vi "Tester_Laser80Calc160.vi"() -> ()   [LabVIEW 2012]
uses:
  <vilib>/Platform/TimedLoop/XDataNode/timing_clust.ctl
  <vilib>/Platform/TimedLoop/XDataNode/nitl_modes.ctl
  <vilib>/Platform/TimedLoop/XDataNode/wakeup.ctl
  <vilib>/rvi/Emulation/niFpgaSctlEmulationRegisterWithScheduler.vi
  <vilib>/rvi/eio/common/nirviEmuTemplateMethod_errors.vi
  <vilib>/rvi/Emulation/niFpgaSctlEmulationScheduler.vi
  <vilib>/rvi/FIFO/Fifo_Resource/nirvififoEmulationSetSize.vi
  <vilib>/rvi/DataTransferAndStorage/Container/Common/niFpgaContainerGetUniqueNameForEmu.vi
  <vilib>/rvi/errors/niFpgaSetErrorForExecOnDevCompSimple.vi
  <vilib>/rvi/eio/common/nirviEmuReportErrorAndStop.vi
  <vilib>/rvi/Emulation/niFpgaSctlEmulationFifoFullMgr.vi
  <vilib>/rvi/Emulation/niFpgaSctlEmulationResourceMgr.vi
  <vilib>/rvi/interface/RandomDataEmulation/nirviRandomDataFPGAFIFO.vi
  <vilib>/rvi/interface/RandomDataEmulation/niFpgaRandomDataHandleErrors.vi
  <vilib>/rvi/Emulation/niFpgaSctlEmulationGlobalWrite.vi
  <vilib>/Platform/TimedLoop/XDataNode/XDataNode.xnode
  <vilib>/eio/EIONode/EIONode.xnode
  <vilib>/rvi/DataTransferAndStorage/Container/XNode/niFpgaContainer.xnode
  <vilib>/rvi/FIFO/Fifo_Resource/nirvififoEmulationClear.vi
  <vilib>/rvi/FIFO/Fifo_Resource/nirvififoEmulationWrite.vi
  <vilib>/rvi/FIFO/Fifo_Resource/nirvififoEmulationRead.vi
  <vilib>/rvi/interface/RandomDataEmulation/nirviRandomDataFpgaReadWriteTemplate.vi
  <vilib>/Platform/TimedLoop/XDataNode/XDNodeRunTimeDep.lvlib
panel:
  out "ToHostAreas FIFO Overflow":bool
  out "ToHostArea1LaserRaw FIFO Overflow":bool
  out "ToHostCh1Raw FIFO Overflow":bool
  out "ToHost FIFO Overflow A1Ch2":bool
  in  "Switch for":i32=6 caption="Requested pixels"
  in  "Laser bitslip":bool
  in  "Laser delay inc":bool
  in  "Samples per pixel Acq A2":u16=10000 caption="Samples per pixel Acq"
  in  "Samples per pixel Acq A1":u16=10000 caption="Samples per pixel Acq"
  in  "Requested pixels A2":u32=100000 caption="Requested pixels"
  in  "Samples per pixel A2":u16=10000 caption="Samples per pixel"
  out "Acquiring":bool
  in  "Wait for trigger":bool
  in  "Acquire continuously":bool=TRUE
  in  "Requested pixels A1":u32=100000 caption="Requested pixels"
  in  "Clear Interloop FIFO":bool
  out "Interloop FIFO overflow":bool
  in  "Samples per pixel A1":u16=10000 caption="Samples per pixel"
  in  "Acquire":bool
  out "Interloop FIFO timeout":bool
  in  "Commit":bool
  out "Xpoint_Switch_Ready":bool
  in  "Xpoint_Switch_Write":bool
  in  "Clock Source":u8(ring)=3 items=["Tristate"=0, "Sync Clock (PXIe only)"=2, "Adapter Module Onboard Clock"=3, "Strobe from Crosspoint Switch"=4, "Strobe Bypass"=5]
  in  "Onboard_Clock_Write":bool
  in  "Onboard_Clock_Write_Data":u16
  out "Onboard_Clock_Ready":bool
  in  "Acq_Reset":bool
  # "6587 IO module configuration"
  # "Tester - Laser80MHz/Calculate 160MHz"
  # "Acquisition control"
  # "Area 1"
  # "Area 2"
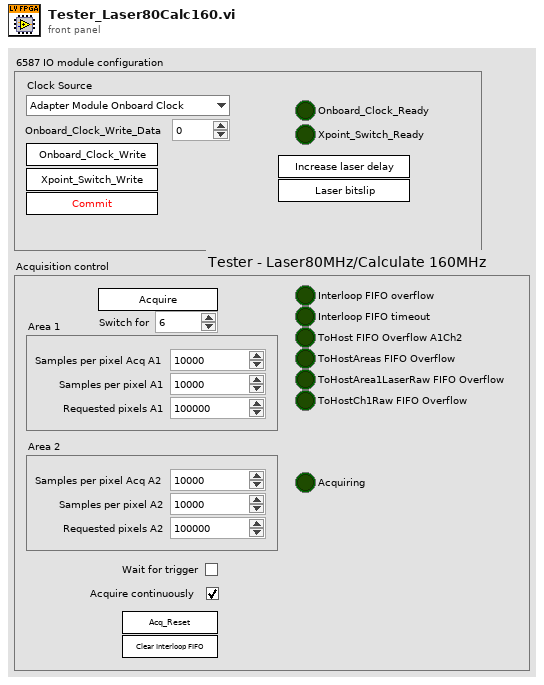
[diagram p1: front panel]
types:
  T1 = typedef "XDNodeRunTimeDep.lvlib/timing_clust.ctl" = cluster{"Expected End [f-1]":u64, "Actual End [f-1]":u64, "Finished Late? [f-1]":bool, "Expected End [i-1]":u64, "Actual End [i-1]":u64, "Finished Late? [i-1]":bool, "Expected Start [i]":u64, "Actual Start [i]":u64, "Expected Start [f]":u64, "Actual Start [f]":u64, "Source Name":string, "Structure Name":string, "Period":i64, "Deadline":i64, "Offset":i64, "Start":i64, "Priority":i32, "Timeout":i32, "Mode":T2, "Wakeup Reason":T3, "Error":errorcluster, "Source Type":string, "Secondary Source Type":string, "Global End Time":u64, "Global Start Time":u64, "Frame Duration":u64, "Iteration Duration":u64, "Assigned CPU":i32, "I/O Scan Engine Mode":u32}
  T2 = typedef "XDNodeRunTimeDep.lvlib/nitl_modes.ctl" = enum32{"No Change", "Process missed periods, maintain original phase", "Discard missed periods, maintain original phase", "Process missed periods, ignore original phase", "Discard missed periods, ignore original phase"}
  T3 = typedef "XDNodeRunTimeDep.lvlib/wakeup.ctl" = enum32{"Normal", "Aborted", "Asynchronous wakeup", "Timing source error", "Timed loop error", "Timeout"}
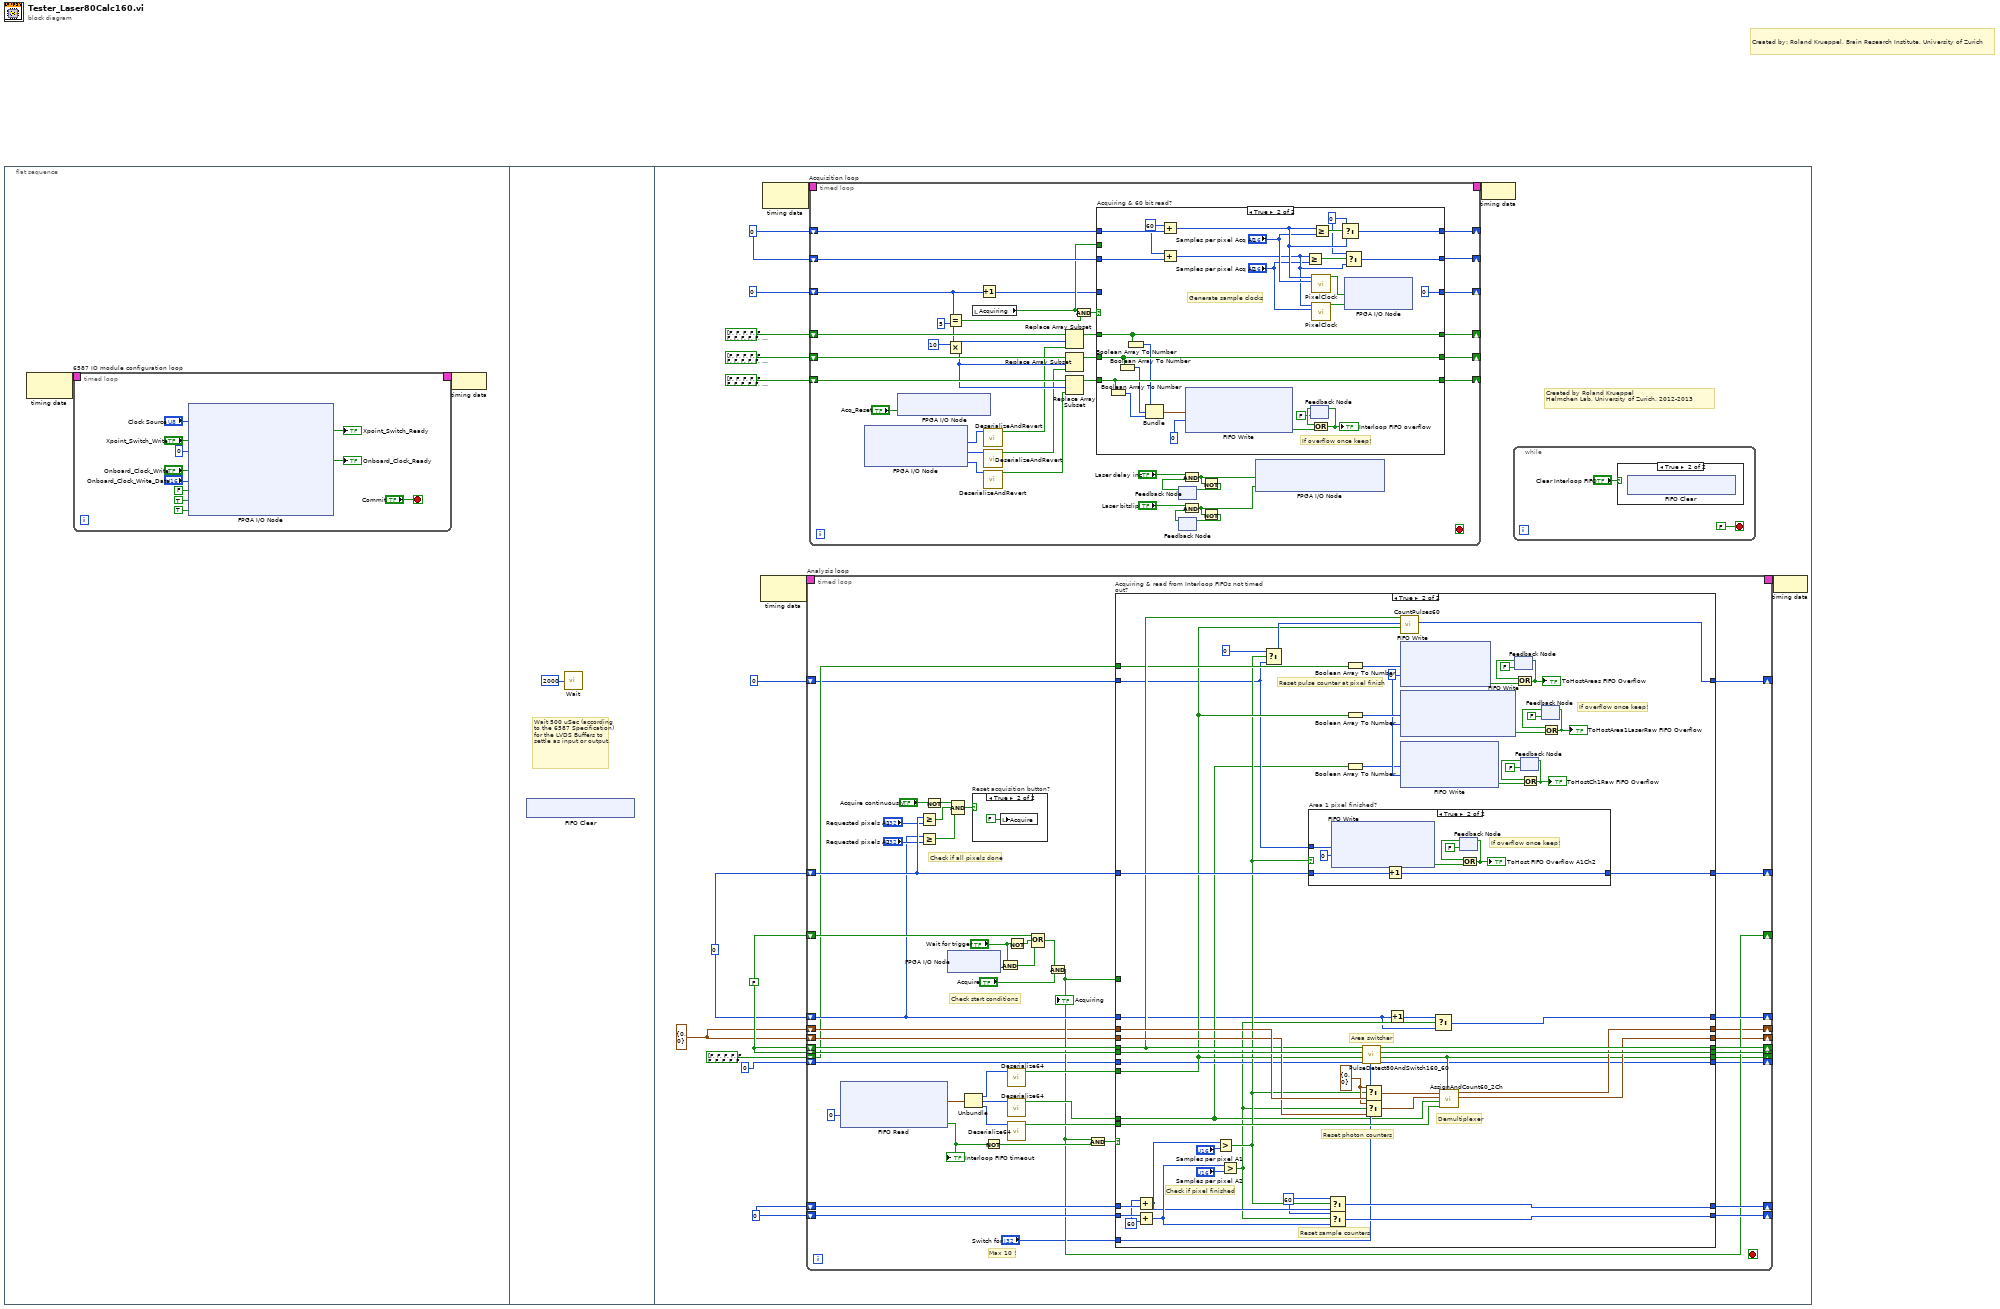
[diagram p0: block diagram]
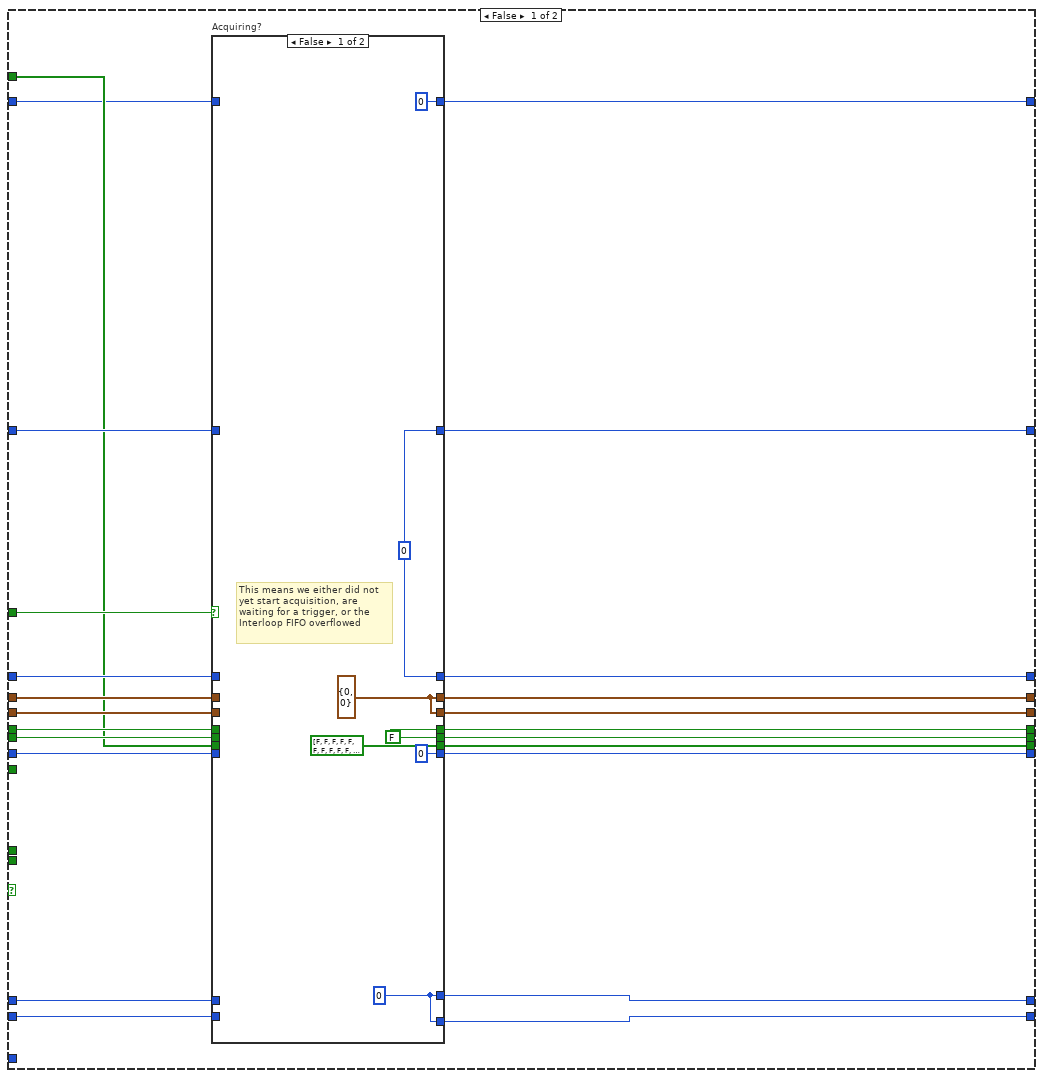
[diagram p4: hidden frame]
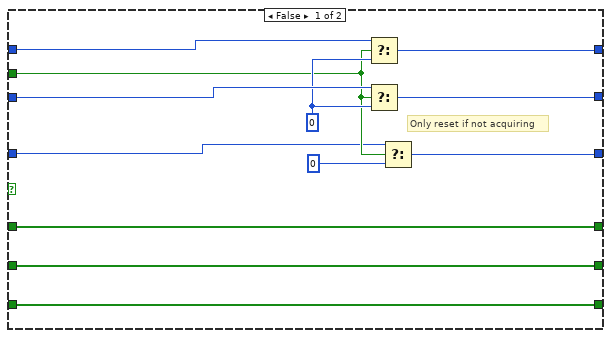
[diagram p7: hidden frame]
diagram:
  # "Created by: Roland Krueppel, Brain Research Institute, University of Zurich"
  n1 = flat-sequence {
    frame #0 {
      n2 = node-c288() -> (w2:T1)  [unwired: 1 in]
      n3 = timed-loop "6587 IO module configuration loop" {
        timing: w2 -> [_]
        timing-out: [_] -> w1
        stop <- "Commit" stop-if-true
        n4 = xnode "FPGA I/O Node"("IO Module\\Acq_IO_Clock_Source"="Clock Source", "IO Module\\Xpoint_Switch_Write"="Xpoint_Switch_Write", "IO Module\\LVDS_Data_Dir"=u16 0 ("IO Module\\LVDS_Data_Dir"), "IO Module\\Onboard_Clock_Write"="Onboard_Clock_Write", "IO Module\\Onboard_Clock_Write_Data"="Onboard_Clock_Write_Data", "IO Module\\SE_PFI0_WE"=FALSE ("IO Module\\SE_PFI0_WE"), "IO Module\\SE_PFI1_WE"=TRUE ("IO Module\\SE_PFI1_WE"), "IO Module\\SE_PFI2_WE"=TRUE ("IO Module\\SE_PFI2_WE")) -> ("IO Module\\Xpoint_Switch_Ready"=→"Xpoint_Switch_Ready":bool, "IO Module\\Onboard_Clock_Ready"=→"Onboard_Clock_Ready":bool)  [unwired: 10 in, 10 out]
      }
      n5 = node-c288(w1) -> ()
    }
    frame #1 {
      # "Wait 500 uSec (according to the 6587 Specification) for the LVDS Buffers to settle as input or output."
      n6 = xnode "FIFO Clear"() -> ()  [unwired: 1 in, 1 out]
      n7 = call "Wait"("Count(uSec)"=u32 2000) -> ()  [unwired: 1 out]
    }
    frame #2 {
      w19 = u16 0 ("t")
      w23 = cluster{u16, u16} {0, 0} ("output cluster")
      w24 = u16 0
      w25 = u32 0 ("Cycle counter out")
      w26 = FALSE ("Last laser bit out")
      # "Created by Roland Krueppel\nHelmchen Lab, University of Zurich, 2012-2013"
      n8 = node-c288() -> (w32:T1)  [unwired: 1 in]
      n9 = node-c288() -> (w34:T1)  [unwired: 1 in]
      n10 = timed-loop "Analysis loop" {
        timing: w32 -> [_]
        timing-out: [_] -> w31
        shift-right: [w82] -> _
        shift-left: w26 -> [w85]
        shift-right: [w84] -> _
        shift-left: w26 -> [w83]
        shift-right: [w58] -> _
        shift-left: w19 -> [w81]
        shift-right: [w56] -> _
        shift-left: w25 -> [w80]
        shift-right: [w54] -> _
        shift-left: w26 -> [w69]
        shift-right: [w57] -> _
        shift-left: w19 -> [w64]
        shift-right: [w55] -> _
        shift-left: w25 -> [w62]
        shift-right: [w45] -> _
        shift-left: w23 -> [w47]
        shift-right: [w44] -> _
        shift-left: w23 -> [w46]
        shift-right: [w43] -> _
        shift-left: bool[] [FALSE, FALSE, FALSE, FALSE, FALSE, FALSE, FALSE, FALSE, FALSE, FALSE, FALSE, FALSE, FALSE, FALSE, FALSE, FALSE, FALSE, FALSE, FALSE, FALSE, FALSE, FALSE, FALSE, FALSE, FALSE, FALSE, FALSE, FALSE, FALSE, FALSE, FALSE, FALSE, FALSE, FALSE, FALSE, FALSE, FALSE, FALSE, FALSE, FALSE, FALSE, FALSE, FALSE, FALSE, FALSE, FALSE, FALSE, FALSE, FALSE, FALSE, FALSE, FALSE, FALSE, FALSE, FALSE, FALSE, FALSE, FALSE, FALSE, FALSE] ("Area bits out") -> [w42]
        shift-right: [w41] -> _
        shift-left: u16 0 ("New pulse count") -> [w40]
        shift-right: [w39] -> _
        shift-left: 0 ("Fill after last") -> [w38]
        stop <- _ stop-if-true
        # "Max 10 !"
        # "Check start conditions"
        # "Check if all pixels done"
        n11 = xnode ("FIFO Read")("Timeout"=0) -> ("Element"=w51:cluster{"Laser":u64, "Ch0":u64, "Ch1":u64}, "Timed Out?"=w52:bool)  [unwired: 1 in, 1 out]
        "Interloop FIFO timeout" <- w52
        n12 = Greater Or Equal?(x=w80, y="Requested pixels A1") -> (x >= y?=w60:bool)
        n13 = Greater Or Equal?(x=w62, y="Requested pixels A2") -> (x >= y?=w59:bool)
        n14 = Not(x="Acquire continuously") -> (.not. x?=w61:bool)
        n15 = xnode "FPGA I/O Node"() -> ("TriggerIn"=w75:bool)  [unwired: 1 in, 1 out]
        n16 = Compound Arithmetic op=AND(w61, w60, w59) -> (w77:bool)
        n17 = Unbundle(w51) -> ("Laser"=w50:u64, "Ch0"=w49:u64, "Ch1"=w48:u64)
        n18 = case "Reset acquisition button?" shown="True" w77 {
          frame False {
          }
          frame True {
            n19 = local write "Acquire"(FALSE ("Acquire")) -> ()
          }
        }
        n20 = Not(x=w52) -> (.not. x?=w70:bool)
        n21 = And(x="Wait for trigger", y=w75) -> (x .and. y?=w72:bool)
        n22 = call "Deserialize64.vi"("U64 input"=w50) -> ("60bit output"=w67:bool[])  [unwired: 10 in]
        n23 = call "Deserialize64.vi"("U64 input"=w49) -> ("60bit output"=w66:bool[])  [unwired: 10 in]
        n24 = call "Deserialize64.vi"("U64 input"=w48) -> ("60bit output"=w65:bool[])  [unwired: 10 in]
        n25 = Not(x="Wait for trigger") -> (.not. x?=w73:bool)
        n26 = Compound Arithmetic op=OR(w69, w73, w72) -> (w71:bool)
        n27 = And(x=w71, y="Acquire") -> (x .and. y?=w54:bool)
        "Acquiring" <- w54
        n28 = And(x=w54, y=w70) -> (x .and. y?=w68:bool)
        n29 = case "Acquiring & read from Interloop FIFOs not timed out?" shown="True" w68 {
          tunnel: w85 -> [w104 w171]
          tunnel: w47 -> [w108 w168]
          tunnel: [w103 w170] -> w84
          tunnel: w83 -> [w105 w159]
          tunnel: [w102 w169] -> w82
          tunnel: w81 -> [w107 w183]
          tunnel: w80 -> [w106 w179]
          tunnel: w67 -> [_ w152]
          tunnel: w66 -> [_ w145]
          tunnel: w54 -> [w109 _]
          tunnel: w65 -> [_ w164]
          tunnel: w64 -> [w96 w181]
          tunnel: w62 -> [w99 w140]
          tunnel: [w97 w173] -> w58
          tunnel: [w95 w175] -> w57
          tunnel: [w101 w162] -> w45
          tunnel: [w100 w178] -> w56
          tunnel: [w98 w141] -> w55
          tunnel: w46 -> [w94 w166]
          tunnel: [w93 w161] -> w44
          tunnel: [w91 w160] -> w43
          tunnel: w42 -> [w92 w154]
          tunnel: [w89 w158] -> w41
          tunnel: w40 -> [w90 w150]
          tunnel: [w87 w149] -> w39
          tunnel: w38 -> [w88 w148]
          tunnel: "Switch for" -> [_ w147]
          frame False {
            n30 = case "Acquiring?" shown="False" w109 {
              tunnel: w108 -> [_ w125]
              tunnel: w107 -> [_ w122]
              tunnel: w106 -> [_ w124]
              tunnel: w105 -> [_ w127]
              tunnel: w104 -> [_ w126]
              tunnel: [w116 w127] -> w103
              tunnel: [w116 w126] -> w102
              tunnel: [w114 w125] -> w101
              tunnel: [w115 w124] -> w100
              tunnel: w99 -> [_ w123]
              tunnel: [w115 w123] -> w98
              tunnel: [w113 w122] -> w97
              tunnel: [w113 w121] -> w95
              tunnel: w96 -> [_ w121]
              tunnel: w94 -> [_ w120]
              tunnel: [w114 w120] -> w93
              tunnel: w92 -> [_ w119]
              tunnel: [bool[] [FALSE, FALSE, FALSE, FALSE, FALSE, FALSE, FALSE, FALSE, FALSE, FALSE, FALSE, FALSE, FALSE, FALSE, FALSE, FALSE, FALSE, FALSE, FALSE, FALSE, FALSE, FALSE, FALSE, FALSE, FALSE, FALSE, FALSE, FALSE, FALSE, FALSE, FALSE, FALSE, FALSE, FALSE, FALSE, FALSE, FALSE, FALSE, FALSE, FALSE, FALSE, FALSE, FALSE, FALSE, FALSE, FALSE, FALSE, FALSE, FALSE, FALSE, FALSE, FALSE, FALSE, FALSE, FALSE, FALSE, FALSE, FALSE, FALSE, FALSE] ("Area bits out") w119] -> w91
              tunnel: w90 -> [_ w118]
              tunnel: [u16 0 ("New pulse count") w118] -> w89
              tunnel: w88 -> [_ w117]
              tunnel: [0 ("Fill after last") w117] -> w87
              frame False {
                w114 = cluster{u16, u16} {0, 0} ("output cluster")
                w115 = u32 0 ("Cycle counter out")
                w113 = u16 0
                w116 = FALSE ("Last laser bit out")
                # "This means we either did not\nyet start acquisition, are\nwaiting for a trigger, or the\nInterloop FIFO overflowed"
              }
              frame True {
                # "This means we are\nreading faster here\nthan acquiring in\nAcquisition loop\n-> keep all values"
              }
            }
          }
          frame True {
            w146 = 0 ("Timeout")
            w163 = cluster{u16, u16} {0, 0} ("t")
            w172 = u16 60 ("t")
            w180 = u16 60
            # "If overflow once keep!"
            # "Reset pulse counter at pixel finish"
            # "Demultiplexer"
            # "Reset photon counters"
            # "Area switcher"
            # "Check if pixel finished"
            # "Reset sample counters"
            n31 = Add(x=w180, y=w183) -> (x+y=w174:u16)
            n32 = Add(x=w181, y=w180) -> (x+y=w176:u16)
            n33 = Greater?(x=w174, y="Samples per pixel A1") -> (0:w151:bool)
            n34 = Greater?(x=w176, y="Samples per pixel A2") -> (0:w143:bool)
            n35 = Select(t=u16 0, s=w151, f=w150) -> (s? t:f=w157:u16)
            n36 = case "Area 1 pixel finished?" shown="True" w151 {
              tunnel: w179 -> [w184 w192]
              tunnel: [w184 w191] -> w178
              tunnel: w150 -> [_ w190]
              frame False {
              }
              frame True {
                # "If overflow once keep!"
                n37 = xnode ("FIFO Write")("Element"=w190, "Timeout"=0) -> ("Timed Out?"=w186:bool)  [unwired: 1 in, 1 out]
                n38 = Increment(x=w192) -> (x+1=w191:u32)
                n39 = feedback #1(FALSE) -> (w188:bool)
                n40 = Or(x=w188, y=w186) -> (x .or. y?=w185:bool)
                "ToHost FIFO Overflow A1Ch2" <- w185
                n41 = feedback-in #1(w185) -> ()
              }
            }
            n42 = Select(t=w172, s=w151, f=w174) -> (s? t:f=w173:u16)
            n43 = Select(t=w172, s=w143, f=w176) -> (s? t:f=w175:u16)
            n44 = Boolean Array To Number(Boolean array=w154) -> (number=w155:u64)
            n45 = Boolean Array To Number(Boolean array=w152) -> (number=w153:u64)
            n46 = Boolean Array To Number(Boolean array=w145) -> (number=w144:u64)
            n47 = call "PulseDetect80AndSwitch160_60.vi"("Switch for"=w147, "Fill from last"=w148, "Laser bits in"=w152, "Last area in"=w171, "Last laser bit in"=w159) -> ("Fill after last"=w149:i32, "Area bits out"=w160:bool[], "New last area out"=w169:bool, "New last laser bit out"=w170:bool)  [unwired: 3 in]
            n48 = Select(t=w163, s=w151, f=w168) -> (s? t:f=w167:cluster{u16, u16})
            n49 = Select(t=w163, s=w143, f=w166) -> (s? t:f=w165:cluster{u16, u16})
            n50 = Increment(x=w140) -> (x+1=w142:u32)
            n51 = call "CountPulses60.vi"("60bit input"=w152, "Previous pulse count"=w157, "Last sample"=w159) -> ("New pulse count"=w158:u16)  [unwired: 7 in, 1 out]
            n52 = xnode ("FIFO Write")("Element"=w155, "Timeout"=w146) -> ("Timed Out?"=w129:bool)  [unwired: 1 in, 1 out]
            n53 = xnode ("FIFO Write")("Element"=w153, "Timeout"=w146) -> ("Timed Out?"=w133:bool)  [unwired: 1 in, 1 out]
            n54 = xnode ("FIFO Write")("Element"=w144, "Timeout"=w146) -> ("Timed Out?"=w136:bool)  [unwired: 1 in, 1 out]
            n55 = Select(t=w142, s=w143, f=w140) -> (s? t:f=w141:u32)
            n56 = call "AssignAndCount60_2Ch.vi"("Area bits in"=w160, "PMT bits Ch2 in"=w164, "PMT bits Ch1 in"=w145, "Photon counters area 2 in"=w165, "Photon counters area 1 in"=w167) -> ("Photon counters area 2 out"=w161:cluster{u16, u16}, "Photon counters area 1 out"=w162:cluster{u16, u16})  [unwired: 5 in]
            n57 = feedback #2(FALSE) -> (w128:bool)
            n58 = Or(x=w128, y=w129) -> (x .or. y?=w130:bool)
            "ToHostAreas FIFO Overflow" <- w130
            n59 = feedback-in #2(w130) -> ()
            n60 = feedback #3(FALSE) -> (w139:bool)
            n61 = Or(x=w139, y=w136) -> (x .or. y?=w137:bool)
            "ToHostCh1Raw FIFO Overflow" <- w137
            n62 = feedback-in #3(w137) -> ()
            n63 = feedback #4(FALSE) -> (w132:bool)
            n64 = Or(x=w132, y=w133) -> (x .or. y?=w134:bool)
            "ToHostArea1LaserRaw FIFO Overflow" <- w134
            n65 = feedback-in #4(w134) -> ()
          }
        }
      }
      n66 = timed-loop "Acquisition loop" {
        timing: w34 -> [_]
        timing-out: [_] -> w33
        shift-right: [w224] -> _
        shift-left: bool[] [FALSE, FALSE, FALSE, FALSE, FALSE, FALSE, FALSE, FALSE, FALSE, FALSE, FALSE, FALSE, FALSE, FALSE, FALSE, FALSE, FALSE, FALSE, FALSE, FALSE, FALSE, FALSE, FALSE, FALSE, FALSE, FALSE, FALSE, FALSE, FALSE, FALSE, FALSE, FALSE, FALSE, FALSE, FALSE, FALSE, FALSE, FALSE, FALSE, FALSE, FALSE, FALSE, FALSE, FALSE, FALSE, FALSE, FALSE, FALSE, FALSE, FALSE, FALSE, FALSE, FALSE, FALSE, FALSE, FALSE, FALSE, FALSE, FALSE, FALSE, FALSE, FALSE, FALSE, FALSE] ("Boolean array") -> [w232]
        shift-right: [w223] -> _
        shift-left: bool[] [FALSE, FALSE, FALSE, FALSE, FALSE, FALSE, FALSE, FALSE, FALSE, FALSE, FALSE, FALSE, FALSE, FALSE, FALSE, FALSE, FALSE, FALSE, FALSE, FALSE, FALSE, FALSE, FALSE, FALSE, FALSE, FALSE, FALSE, FALSE, FALSE, FALSE, FALSE, FALSE, FALSE, FALSE, FALSE, FALSE, FALSE, FALSE, FALSE, FALSE, FALSE, FALSE, FALSE, FALSE, FALSE, FALSE, FALSE, FALSE, FALSE, FALSE, FALSE, FALSE, FALSE, FALSE, FALSE, FALSE, FALSE, FALSE, FALSE, FALSE, FALSE, FALSE, FALSE, FALSE] ("Boolean array") -> [w231]
        shift-right: [w222] -> _
        shift-left: 0 -> [w221]
        shift-right: [w217] -> _
        shift-left: bool[] [FALSE, FALSE, FALSE, FALSE, FALSE, FALSE, FALSE, FALSE, FALSE, FALSE, FALSE, FALSE, FALSE, FALSE, FALSE, FALSE, FALSE, FALSE, FALSE, FALSE, FALSE, FALSE, FALSE, FALSE, FALSE, FALSE, FALSE, FALSE, FALSE, FALSE, FALSE, FALSE, FALSE, FALSE, FALSE, FALSE, FALSE, FALSE, FALSE, FALSE, FALSE, FALSE, FALSE, FALSE, FALSE, FALSE, FALSE, FALSE, FALSE, FALSE, FALSE, FALSE, FALSE, FALSE, FALSE, FALSE, FALSE, FALSE, FALSE, FALSE, FALSE, FALSE, FALSE, FALSE] ("Boolean array") -> [w220]
        shift-right: [w215] -> _
        shift-left: w24 -> [w216]
        shift-right: [w213] -> _
        shift-left: w24 -> [w214]
        stop <- _ stop-if-true
        n67 = xnode "FPGA I/O Node"() -> ("IO Module\\LVDS_Ch0_Rd"=w210:u16, "IO Module\\LVDS_Ch1_Rd"=w208:u16, "IO Module\\LVDS_Ch2_Rd"=w206:u16)  [unwired: 3 in, 3 out]
        n68 = xnode "FPGA I/O Node"("IO Module\\Acq_Reset"="Acq_Reset") -> ()  [unwired: 1 in, 1 out]
        n69 = Equal?(x=w221, y=5) -> (x = y?=w228:bool)
        n70 = Multiply(x=10 ("y"), y=w221) -> (x*y=w219:i32)
        n71 = local read "Acquiring"() -> (w212:bool)
        n72 = Increment(x=w221) -> (x+1=w211:i32)
        n73 = call "DeserializeAndRevert.vi"("U16 input"=w210) -> ("10bit output"=w209:bool[])  [unwired: 10 in]
        n74 = call "DeserializeAndRevert.vi"("U16 input"=w208) -> ("10bit output"=w207:bool[])  [unwired: 10 in]
        n75 = call "DeserializeAndRevert.vi"("U16 input"=w206) -> ("10bit output"=w205:bool[])  [unwired: 10 in]
        n76 = Replace Array Subset(array=w232, new element=w209, index=w219) -> (w226:bool[])
        n77 = Replace Array Subset(array=w231, new element=w207, index=w219) -> (w225:bool[])
        n78 = Replace Array Subset(array=w220, new element=w205, index=w219) -> (w218:bool[])
        n79 = And(x=w212, y=w228) -> (x .and. y?=w227:bool)
        n80 = case "Acquiring & 60 bit read?" shown="True" w227 {
          tunnel: w226 -> [w245 w269]
          tunnel: w225 -> [w244 w271]
          tunnel: [w245 w269] -> w224
          tunnel: [w244 w271] -> w223
          tunnel: [w235 0] -> w222
          tunnel: w211 -> [w236 _]
          tunnel: w218 -> [w243 w270]
          tunnel: [w243 w270] -> w217
          tunnel: w216 -> [w242 w268]
          tunnel: [w241 w266] -> w215
          tunnel: w214 -> [w240 w262]
          tunnel: [w239 w258] -> w213
          tunnel: w212 -> [w237 _]
          frame False {
            w238 = u16 0 ("f")
            # "Only reset if not acquiring"
            n81 = Select(t=w242, s=w237, f=w238) -> (s? t:f=w241:u16)
            n82 = Select(t=w240, s=w237, f=w238) -> (s? t:f=w239:u16)
            n83 = Select(t=w236, s=w237, f=0) -> (s? t:f=w235:i32)
          }
          frame True {
            w259 = u16 0 ("t")
            w261 = u16 60 ("x")
            # "If overflow once keep!"
            # "Generate sample clocks"
            n84 = Boolean Array To Number(Boolean array=w270) -> (number=w252:u64)
            n85 = Boolean Array To Number(Boolean array=w271) -> (number=w253:u64)
            n86 = Boolean Array To Number(Boolean array=w269) -> (number=w254:u64)
            n87 = Bundle(w254, w253, w252) -> (w251:cluster{u64, u64, u64})  [unwired: 1 in]
            n88 = Add(x=w261, y=w268) -> (x+y=w265:u16)
            n89 = Add(x=w261, y=w262) -> (x+y=w257:u16)
            n90 = xnode ("FIFO Write")("Element"=w251, "Timeout"=0) -> ("Timed Out?"=w247:bool)  [unwired: 1 in, 1 out]
            n91 = Greater Or Equal?(x=w257, y="Samples per pixel Acq A2") -> (x >= y?=w260:bool)
            n92 = feedback #5(FALSE) -> (w249:bool)
            n93 = call "PixelClock.vi"("Samples per pixel"="Samples per pixel Acq A1", "Sample counter"=w265) -> ("Pixel clock"=w263:bool)  [unwired: 9 in]
            n94 = call "PixelClock.vi"("Samples per pixel"="Samples per pixel Acq A2", "Sample counter"=w257) -> ("Pixel clock"=w255:bool)  [unwired: 9 in]
            n95 = Or(x=w249, y=w247) -> (x .or. y?=w246:bool)
            "Interloop FIFO overflow" <- w246
            n96 = feedback-in #5(w246) -> ()
            n97 = Greater Or Equal?(x=w265, y="Samples per pixel Acq A1") -> (x >= y?=w267:bool)
            n98 = Select(t=w259, s=w267, f=w265) -> (s? t:f=w266:u16)
            n99 = Select(t=w259, s=w260, f=w257) -> (s? t:f=w258:u16)
            n100 = xnode "FPGA I/O Node"("Pixel clock A1"=w263, "Pixel clock A2"=w255) -> ()  [unwired: 2 in, 2 out]
          }
        }
        n101 = feedback #6() -> (w203:bool)  [unwired: 1 in]
        n102 = feedback #7() -> (w198:bool)  [unwired: 1 in]
        n103 = And(x="Laser delay inc", y=w203) -> (x .and. y?=w201:bool)
        n104 = And(x="Laser bitslip", y=w198) -> (x .and. y?=w197:bool)
        n105 = Not(x=w201) -> (.not. x?=w202:bool)
        n106 = feedback-in #6(w202) -> ()
        n107 = Not(x=w197) -> (.not. x?=w200:bool)
        n108 = feedback-in #7(w200) -> ()
        n109 = xnode "FPGA I/O Node"("IO Module\\Ch0_Idelay_Increment"=w201, "IO Module\\Ch0_Bitslip"=w197) -> ()  [unwired: 2 in, 2 out]
      }
      n110 = node-c288(w33) -> ()
      n111 = while {
        stop <- FALSE stop-if-true
        n112 = case shown="True" "Clear Interloop FIFO" {
          frame False {
          }
          frame True {
            n113 = xnode ("FIFO Clear")() -> ()  [unwired: 1 in, 1 out]
          }
        }
      }
      n114 = node-c288(w31) -> ()
    }
  }
